vi "InitPluginPaths.vi"(5 "BusIndex":i32, 7 "PluginIndex":u32[](array[numeric]), 8 "Error In":errorcluster[](array[cluster]), 10 "Modules":string[](array[string]), 11 "Bus in":refnum<class "Bus.lvclass">) -> (0 "Error Out":errorcluster[](array[cluster]), 3 "Bus out":refnum<class "Bus.lvclass">)   [LabVIEW 2018, in "Bus.lvclass"]
uses:
  Bus.lvclass
  Bus.lvclass/Bus.ctl
  TestClass/Test.lvclass/Test.ctl
  TestClass/Accessors/Write PluginIndex.vi
  TestClass/Accessors/Write PluginPathArray.vi
  Accessors/Read Test.vi
  Accessors/Write Test.vi
  <vilib>/Utility/error.llb/Error Cluster From Error Code.vi
  TestClass/Test.lvclass
  <vilib>/ErrorRing/Error Ring.xnode
  LV_Ini/Ini_lib.lvlib
  <userlib>/NIST/NISTErrorLib/NISTErrorLib.lvlib
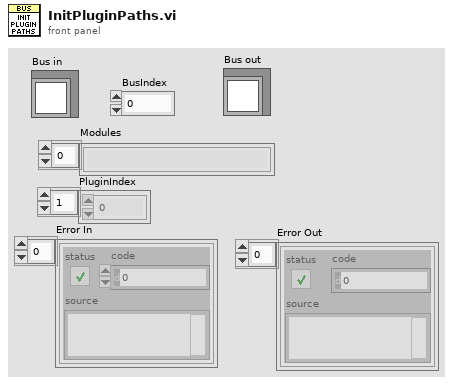
[diagram p1: front panel]
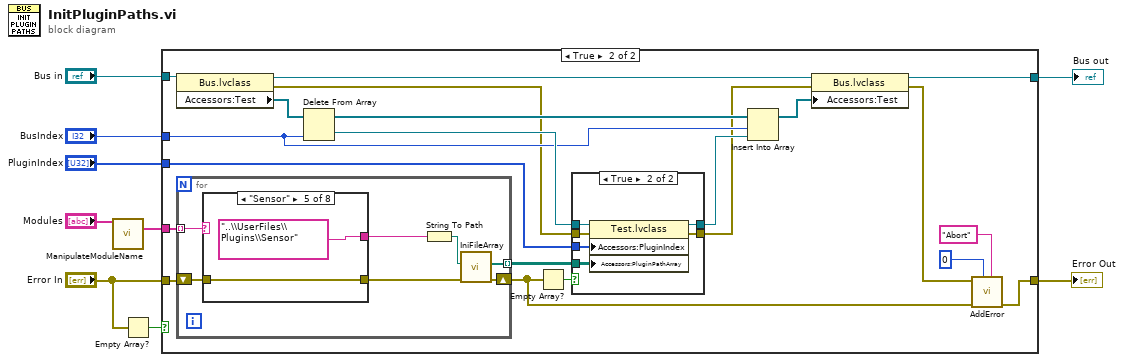
[diagram p0: block diagram]
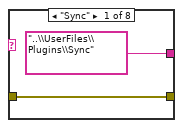
[diagram p4: hidden frame]
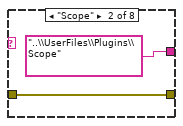
[diagram p5: hidden frame]
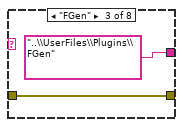
[diagram p6: hidden frame]
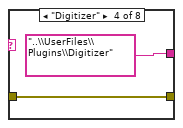
[diagram p7: hidden frame]
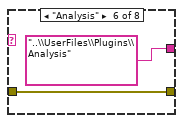
[diagram p8: hidden frame]
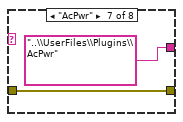
[diagram p9: hidden frame]
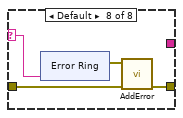
[diagram p10: hidden frame]
diagram:
  n1 = call "ManipulateModuleName.vi"("ModuleListArrayIn"="Modules") -> ("BeforeMatch:ModuleListArray"=w1:string[])  [unwired: 9 in, 5 out]
  n2 = Empty Array?(array="Error In") -> (empty?=w9:bool)
  n3 = case shown="True" w9 {
    tunnel: "Error In" -> [w10 w22]
    tunnel: "Bus in" -> [w11 w30]
    tunnel: [w11 w21] -> w6
    tunnel: [w10 w15] -> w5
    tunnel: "BusIndex" -> [_ w25]
    tunnel: w1 -> [_ w29]
    tunnel: "PluginIndex" -> [_ w19]
    frame False {
    }
    frame True {
      n4 = property class="Bus.lvclass"(reference=w30) -> (reference out=w24:refnum<class "Bus.lvclass">, error out=w13:errorcluster, "Accessors:Test"=w31:refnum<class "Test.lvclass">[])  [unwired: 1 in]
      n5 = for {
        shift-right: [w46] -> w16
        shift-left: w22 -> [w44]
        tunnel: w29 -> [w47] mode=indexing
        tunnel: [w45] -> w28 mode=indexing
        n6 = case shown="\"Sensor\"" w47 {
          selector: w47 -> [_ _ _ _ _ _ _ w64]
          tunnel: ["..\\UserFiles\\Plugins\\Sync" "..\\UserFiles\\Plugins\\Scope" "..\\UserFiles\\Plugins\\FGen" "..\\UserFiles\\Plugins\\Digitizer" "..\\UserFiles\\Plugins\\Sensor" "..\\UserFiles\\Plugins\\Analysis" "..\\UserFiles\\Plugins\\AcPwr" _] -> w41
          tunnel: w44 -> [w48 w50 w52 w54 w56 w58 w60 w65]
          tunnel: [w48 w50 w52 w54 w56 w58 w60 w62] -> w43
          frame "Sync" {
          }
          frame "Scope" {
          }
          frame "FGen" {
          }
          frame "Digitizer" {
          }
          frame "Sensor" {
          }
          frame "Analysis" {
          }
          frame "AcPwr" {
          }
          frame Default {
            n7 = xnode "Error Ring"("parameter 0"=w64) -> ("error out"=w63:errorcluster)
            n8 = call <userlib>:"AddError.vi"("ErrorArray In"=w65, "error in (no error)"=w63) -> ("ErrorArray Out"=w62:errorcluster[])  [unwired: 8 in, 1 out]
          }
        }
        n9 = String To Path(string=w41) -> (path=w42:path)
        n10 = call "IniFileArray.vi"("ErrorArray In"=w43, "Relative Path to Plugins"=w42) -> ("ErrorArray Out"=w46:errorcluster[], "INIFilePaths"=w45:path[])  [unwired: 8 in]
      }
      n11 = Delete From Array(array=w31, index=w25) -> (deleted portion=w32:refnum<class "Test.lvclass">, array with subset deleted=w27:refnum<class "Test.lvclass">[])  [unwired: 1 in]
      n12 = Empty Array?(array=w16) -> (empty?=w20:bool)
      n13 = case shown="True" w20 {
        tunnel: w32 -> [w34 w40]
        tunnel: w28 -> [_ w38]
        tunnel: [w34 w39] -> w26
        tunnel: w19 -> [_ w37]
        tunnel: w13 -> [w33 w36]
        tunnel: [w33 w35] -> w12
        frame False {
        }
        frame True {
          n14 = property class="Test.lvclass"(reference=w40, error in=w36, "Accessors:PluginIndex"=w37, "Accessors:PluginPathArray"=w38) -> (reference out=w39:refnum<class "Test.lvclass">, error out=w35:errorcluster)
        }
      }
      n15 = Insert Into Array(array=w27, index=w25, new element=w26) -> (w23:refnum<class "Test.lvclass">[])
      n16 = property class="Bus.lvclass"(reference=w24, error in=w12, "Accessors:Test"=w23) -> (reference out=w21:refnum<class "Bus.lvclass">, error out=w14:errorcluster)
      n17 = call <userlib>:"AddError.vi"("Severity"="Abort", "Priority"=u8 0, "ErrorArray In"=w16, "error in (no error)"=w14) -> ("ErrorArray Out"=w15:errorcluster[])  [unwired: 6 in, 1 out]
    }
  }
  "Bus out" <- w6
  "Error Out" <- w5
